vi "Array Parameter Support Demo.vi"() -> ()   [LabVIEW 2014]
uses:
  Array-Parameter/_support/Operation-FGV-MassData.ctl
  Array-Parameter/JKISM++ Array Parameter Support.lvlib
panel:
  in  "stop":bool
  out "Thermometer":cluster{dbl, dbl}(slide)={0.0, 6224.489795918367} scale=0.0..1000000.0 scale format="%#_6p"
  out "Argument":string
  out "Waveform Graph":dbl[](graph)
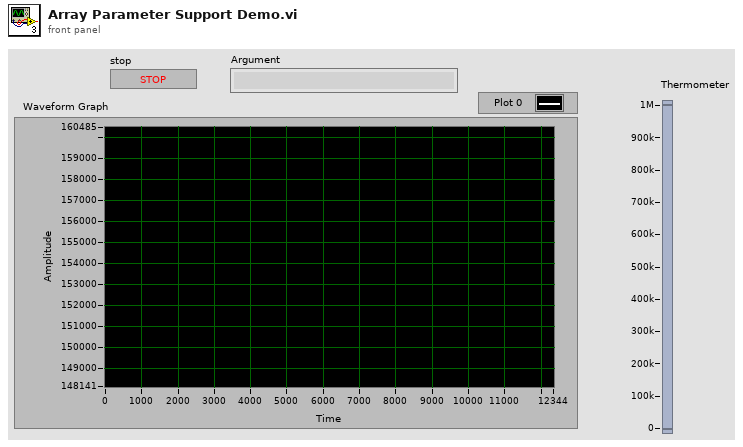
[diagram p1: front panel]
types:
  T1 = typedef "JKISM++ Array Parameter Support.lvlib/Operation-FGV-MassData.ctl" = enum16{"Initialize", "Read", "Write", "Status", "Release"}
  T2 = typedef "JKISM++ Array Parameter Support.lvlib/Def-MassDataOper-Status.ctl" = cluster{"Start":i32, "Size":i32, "Total":i32}
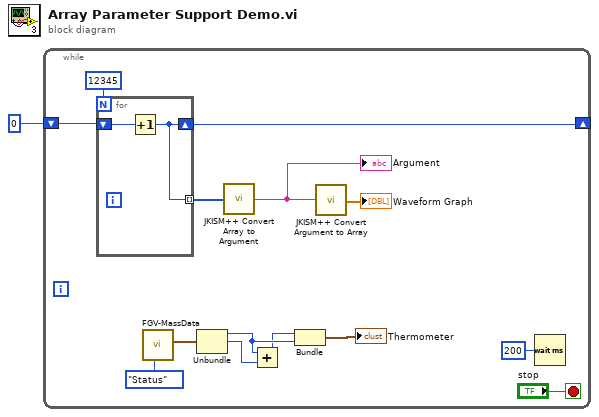
[diagram p0: block diagram]
diagram:
  n1 = while {
    shift-right: [w2] -> _
    shift-left: 0 -> [w3]
    stop <- "stop" stop-if-true
    n2 = for {
      N: 12345 -> [_]
      tunnel: [w16] -> w13 mode=indexing
      shift-right: [w16] -> w2
      shift-left: w3 -> [w17]
      n3 = Increment(x=w17) -> (x+1=w16:i32)
    }
    n4 = call "FGV-MassData.vi"("Operation"=Operation-FGV-MassData."Status") -> ("Active Write Oper"=w6:T2)  [unwired: 7 in, 3 out]
    n5 = Unbundle(w6) -> ("Start"=w9:i32, "Size"=w7:i32)  [unwired: 1 out]
    n6 = call "JKISM++ Convert Array to Argument.vi"("DBL"=w13) -> ("Argument"=w15:string)  [unwired: 8 in]
    "Argument" <- w15
    n7 = Add(x=w9, y=w7) -> (x+y=w8:i32)
    n8 = Bundle(w8, "Start"=w9) -> (→"Thermometer":cluster{i32, "Start":i32})  [unwired: 1 in]
    n9 = call "JKISM++ Convert Argument to Array.vi"("HEX Argument"=w15) -> ("DBL"=→"Waveform Graph":dbl[])  [unwired: 8 in]
    n10 = Wait (ms)(milliseconds to wait=u32 200) -> ()  [unwired: 1 out]
  }
